vi "fgt close.vi"(8 "error in (no error)":errorcluster) -> (0 "error out":errorcluster)   [LabVIEW 2020, in "fgt_SDK.lvlib"]
doc: "Close communication with Fluigent instruments and free memory.\nThis function is mandatory, if not called the dll will be automatically closed when exiting your application.\nUsing this function will remove session preferences such as units and limits. If any regulation is running it will stop pressure control."
uses:
  fgt_SDK.lvlib
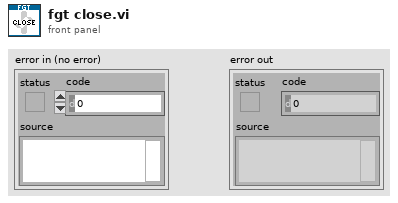
[diagram p1: front panel]
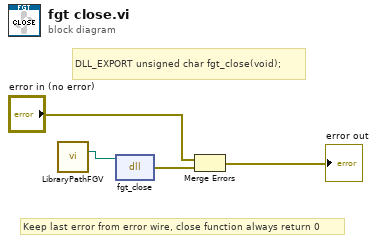
[diagram p0: block diagram]
diagram:
  # "Keep last error from error wire, close function always return 0"
  # "DLL_EXPORT unsigned char fgt_close(void);"
  n1 = call "LibraryPathFGV.vi"() -> ("Path Out"=w1:path)  [unwired: 14 in, 1 out]
  n2 = dll-call lib="C:/Workspace/fgt-SDK/LabVIEW/dlls/fgt_SDK_*.*" fn="fgt_close"(path in=w1) -> (error out=w4:errorcluster)  [unwired: 3 in, 1 out]
  n3 = Merge Errors("error in (no error)", w4) -> (→"error out":errorcluster)
